vi "PS_COND+TEMP.vi"(0 "GUID":string) -> (1 "Ohms":dbl, 3 "File Path Out":path[](array[path]), 4 "VI-time":dbl, 5 "Cell_Constant":dbl=0.33, 6 "Cond (mS)":dbl, 7 "Temp (C)":dbl, 8 "Temp_Calib_Offset":dbl=4.8, 9 "time date":string, 10 "Hz":dbl)   [LabVIEW 2019]
uses:
  5_Controls/PS_CMD_type-def.ctl
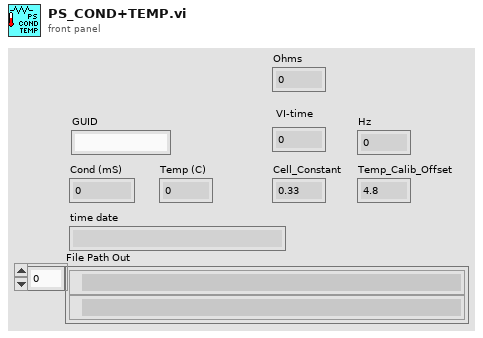
[diagram p1: front panel]
types:
  T1 = typedef "PS_CMD_type-def.ctl" = enum16{"Cond+Temp", "Cond_EIS", "Temp_EIS", "Vwind_MSP", "LongCond", "Cell1_EIS", "Cell2_EIS", "Cell3_EIS"}
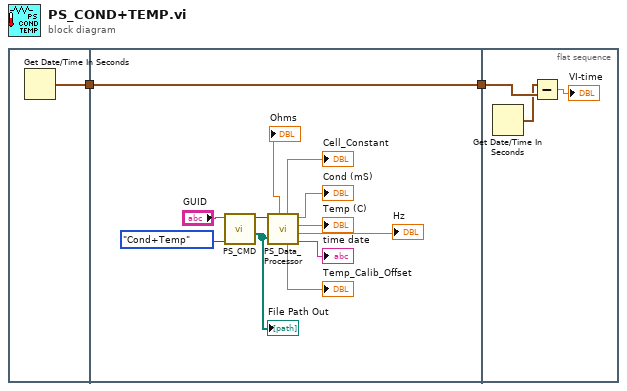
[diagram p0: block diagram]
diagram:
  n1 = flat-sequence {
    tunnel: [w3] -> w1
    tunnel: [w8] -> w2
    tunnel: w1 -> [w8]
    tunnel: w2 -> [w18]
    frame #0 {
      n2 = Get Date/Time In Seconds() -> (seconds since 1Jan1904=w3:timestamp)
    }
    frame #1 {
      n3 = call "PS_CMD.vi"(4:PS_CMD_type-def."Cond+Temp", "GUID"="GUID") -> ("File Path Out"=w13:path[], "Enum"=w14:T1)  [unwired: 4 in]
      "File Path Out" <- w13
      n4 = call "PS_Data_Processor.vi"("file path (dialog if empty)"=w13, 11:w14) -> ("time date"=→"time date":string, "Hz"=→"Hz":dbl, "Cond (mS)"=→"Cond (mS)":dbl, "TempCalibOffset 2"=→"Temp_Calib_Offset":dbl, "Cell Constant 2"=→"Cell_Constant":dbl, "Ohms"=→"Ohms":dbl, "Temp (C)"=→"Temp (C)":dbl)  [unwired: 2 in, 1 out]
    }
    frame #2 {
      n5 = Get Date/Time In Seconds() -> (seconds since 1Jan1904=w17:timestamp)
      n6 = Subtract(x=w17, y=w18) -> (x-y=→"VI-time":dbl)
    }
  }
